vi "EF_GetFeaturesVectorBicoherence.vi"(8 "error in (no error)":errorcluster, 9 "High cutoff frequency":dbl, 10 "Low cutoff frequency":dbl, 11 "Array Of Waveforms in":waveform(dbl)[](array[waveform])) -> (0 "error out":errorcluster, 3 "Bicoherence features out":dbl[][](array[numeric]))   [LabVIEW 2016, in "Feature Extraction.lvlib"]
uses:
  <vilib>/addons/Time Series Analysis/Correlation and Spectral Analysis.llb/TSA Bicoherence (Waveform).vi
  Feature Extraction.lvlib
  <vilib>/addons/_Advanced Signal Processing/NI_AdvSigProcTSA.lvlib
panel:
  out "Сигнал ЭЭГ":waveform(dbl)(graph)
  out "Матрица коэффициентов биспектра":dbl[][](graph)
  # "This VI is a part of BCI Design library, http://www.ru-bci.org \nCopyright © 2020, Sotnikov Peter, All rights reserved. License: GNU GPLv3"
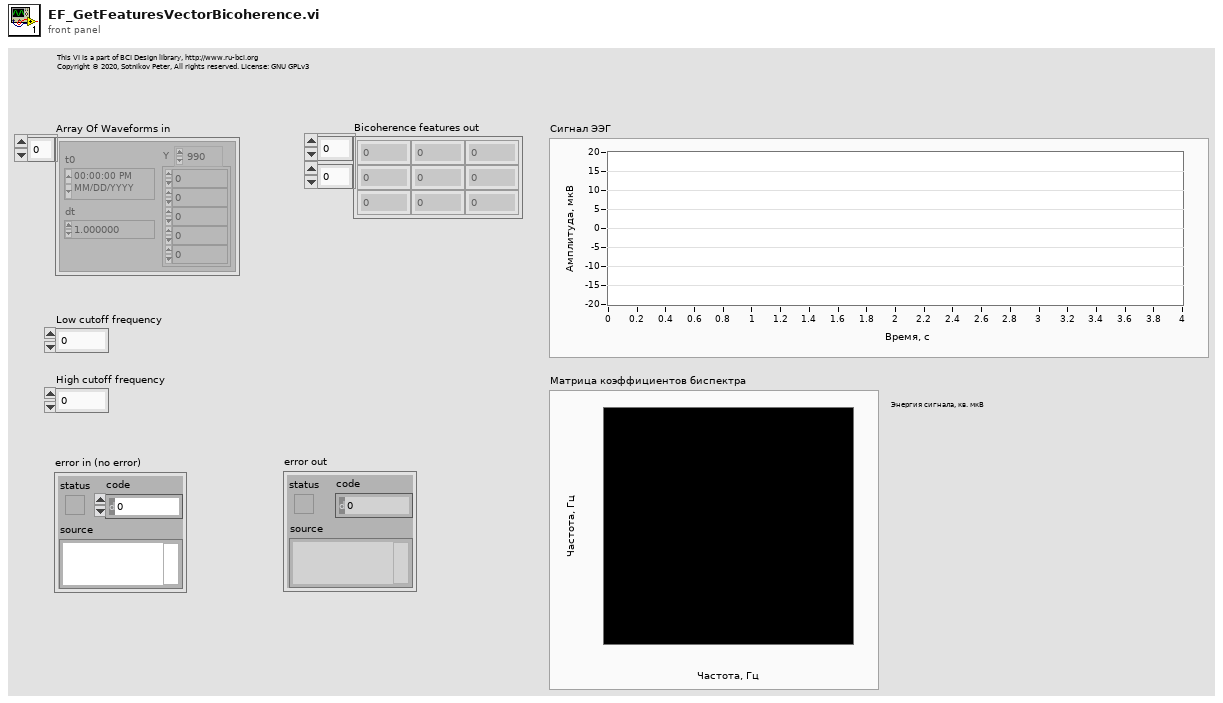
[diagram p1: front panel]
types:
  T1 = cluster{"window":u16, "length":i32, "overlap (%)":dbl}
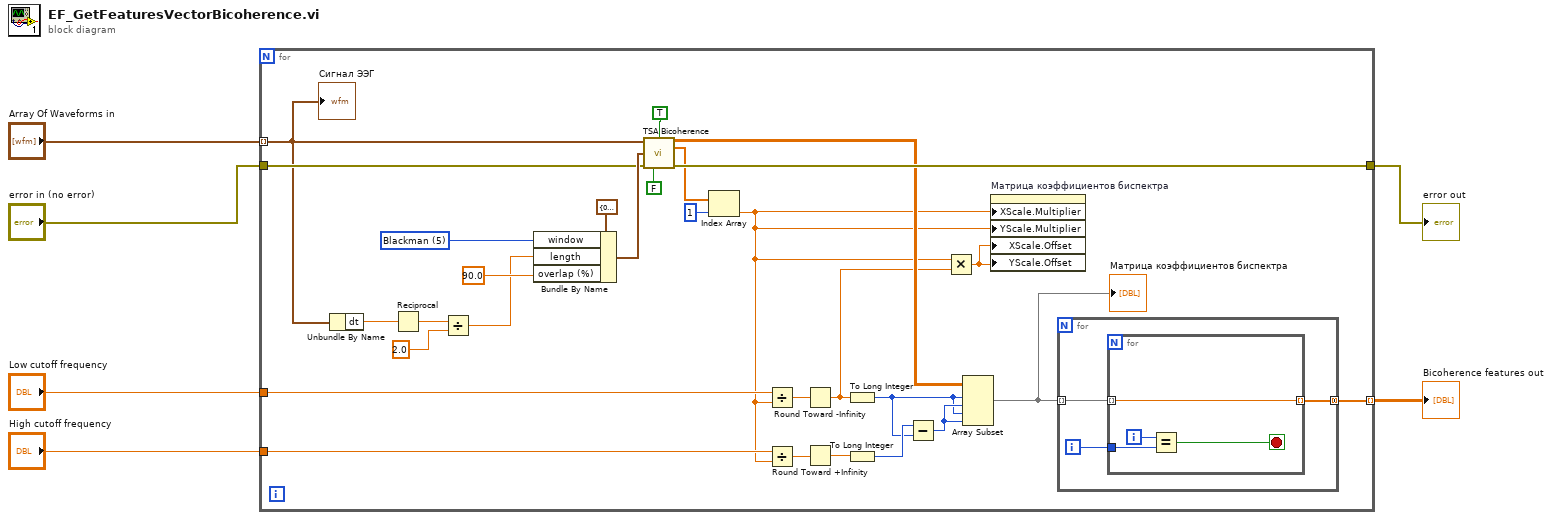
[diagram p0: block diagram]
diagram:
  n1 = for {
    tunnel: "Array Of Waveforms in" -> [w8] mode=indexing
    tunnel: "error in (no error)" -> [w27]
    tunnel: "Low cutoff frequency" -> [w21]
    tunnel: "High cutoff frequency" -> [w20]
    tunnel: [w28] -> w2
    tunnel: [w9] -> w1 mode=indexing
    w31 = u16 5 items=["None ", "Hanning", "Hamming", "Blackman-Harris", "Exact Blackman", "Blackman", "Flat Top", "4 Term B-Harris ", "7 Term B-Harris", "Low Sidelobe"] ("window")
    n2 = Unbundle By Name(w8) -> ("dt"=w29:dbl)
    n3 = Reciprocal(x=w29) -> (1/x=w26:dbl)
    n4 = Divide(x=w26, y=2.0) -> (x/y=w25:dbl)
    n5 = Bundle By Name(cluster=T1 {"window"=0, "length"=-1, "overlap (%)"=50.0} ("window info"), "window"=w31, "length"=w25, "overlap (%)"=90.0) -> (w32:T1)
    n6 = call-poly <vilib>:"TSA Bicoherence.vi"("Xt"=w8, "initialize? (F)"=TRUE, "window info"=w32, "error in (no error)"=w27, "dB on? (T)"=FALSE) -> ("S(f,f)"=w18:dbl[][], "freq bins"=w23:dbl[], "error out"=w28:errorcluster)  [unwired: 8 in]
    n7 = Index Array(array=w23, index=1) -> (element=w12:dbl)
    n8 = Divide(x=w21, y=w12) -> (x/y=w16:dbl)
    n9 = Divide(x=w20, y=w12) -> (x/y=w15:dbl)
    n10 = Round Toward -Infinity(1:w16) -> (0:w10:dbl)
    n11 = Round Toward +Infinity(x=w15) -> (ceil(x): smallest int >= x=w14:dbl)
    n12 = To Long Integer(number=w10) -> (32bit integer=w13:i32)
    n13 = To Long Integer(number=w14) -> (32bit integer=w19:i32)
    n14 = Subtract(x=w19, y=w13) -> (x-y=w17:i32)
    n15 = Multiply(x=w12, y=w10) -> (x*y=w11:dbl)
    n16 = Array Subset(array=w18, index (row)=w13, length (row)=w17, index (col)=w13, length (col)=w17) -> (w7:dbl[][])
    "Матрица коэффициентов биспектра" <- w7
    n17 = property on="Матрица коэффициентов биспектра" class="IntGraph (strict)"("XScale.Multiplier"=w12, "YScale.Multiplier"=w12, "XScale.Offset"=w11, "YScale.Offset"=w11) -> ()  [unwired: 2 in, 2 out]
    n18 = for {
      tunnel: w7 -> [w38] mode=indexing
      tunnel: [w36] -> w9 mode=concatenating
      i -> [w37]
      n19 = for {
        tunnel: w38 -> [w39] mode=indexing
        tunnel: w37 -> [w41]
        tunnel: [w39] -> w36 mode=indexing
        i -> [w42]
        stop <- w40 stop-if-true
        n20 = Equal?(x=w42, y=w41) -> (x = y?=w40:bool)
      }
    }
    "Сигнал ЭЭГ" <- w8
  }
  "error out" <- w2
  "Bicoherence features out" <- w1
